vi "Configuration Parse.vi"(8 "error in":errorcluster, 11 "Measurement Configuration":T1={"Automation Test"=FALSE, "Power sequencing file path"="", "VST Resource Name"="5842", "RFSG port"="Port1", "RFmx port"="Port2", "RF Out Switch"="2599_S8", "Common RFout"="COM0", "Port1 Incident"="NC0", "Port2 Incident"="NO0", "RF In Switch"="2597_S12", "Common RFin"="COM", "Port1 Reference"="CH1", "Port1 Test"="CH2", "Port2 Reference"="CH4", "Port2 Test"="CH3", "RFSG attenuation mode"=enum."<None>", "RFSG external attenuation (dB)"=0.0, "Save Calibration File at"="", "Short S1P"="", "Open S1P"="", "Load S1P"="", "Through Adapter S2P"="", "Action"=enum."Measure", "Power Level (dBm)"=0.0, "External Gain (dB)"=-6.0, "Start Frequency (Hz)"=6000000000.0, "Stop Frequency (Hz)"=12000000000.0, "Step Size (Hz)"=100000000.0, "Type of Stimulus"=enum."CW", "Pulse Width (s)"=0.0, "PRI (s)"=0.0, "IF Bandwidth (Hz)"=10000.0, "Average Mode"=enum."Per Sweep", "Number of Averages"=1, "SnP File Path"="", "Calibration File Path"="", "Power sequecing file validity check"=TRUE} {"Step Size (Hz)" format="%#_6p"; "Stop Frequency (Hz)" format="%.3p"; "Start Frequency (Hz)" format="%.3p"; "Power Level (dBm)" format="%.2f"; "RFSG external attenuation (dB)" format="%.2f"}) -> (0 "error out":errorcluster, 2 "RFmxVNA Settings":T3={"VST Resource Name"="VNA-5633", "RFSG Port"="", "RFmx Port"="", "RF Out Switch"="VNA-5633", "RF Out Connection"={"Common RFout"="", "Port1 Incident"="", "Port2 Incident"=""}, "RF In Switch"="VNA-5633", "RF In Connection"={"Common RFin"="", "Port1 Reference"="", "Port1 Test"="", "Port2 Reference"="", "Port2 Test"=""}, "RFSG attenuation mode"=enum."Constant Attenuation", "RFSG Constant Attenuation (dB)"=0.0, "Save Calibration File at"=path "", "Short S1P"=path "", "Open S1P"=path "", "Load S1P"=path "", "Through Adapter S2P"=path ""}, 3 "Test Configuration":T2={"Action"=enum."Measure", "Power Level (dBm)"=0.0, "External Gain (dB)"=0.0, "Frequency Sweep"={"Start Frequency (Hz)"=0.0, "Stop Frequency (Hz)"=0.0, "Step Size (Hz)"=0.0}, "Type of Stimulus"=enum."CW", "Pulse Width (s)"=0.0, "PRI (s)"=0.0, "IF Bandwidth (Hz)"=0.0, "Average Mode"=enum."Per Sweep", "Number of Averages"=0, "SnP File Path"=path "", "Calibration File Path"=path ""} {"Frequency Sweep"."Step Size (Hz)" format="%#_6p"; "Frequency Sweep"."Stop Frequency (Hz)" format="%.3p"; "Frequency Sweep"."Start Frequency (Hz)" format="%.3p"})   [LabVIEW 2023, in "FPT_SParam_VST.lvclass"]
uses:
  FPT_SParam_VST.lvclass
  Measurement/Controls/Hardware Config - SParam_VST.ctl
  Measurement/Controls/Test Config - SParam_VST.ctl
  Measurement Configuration.ctl
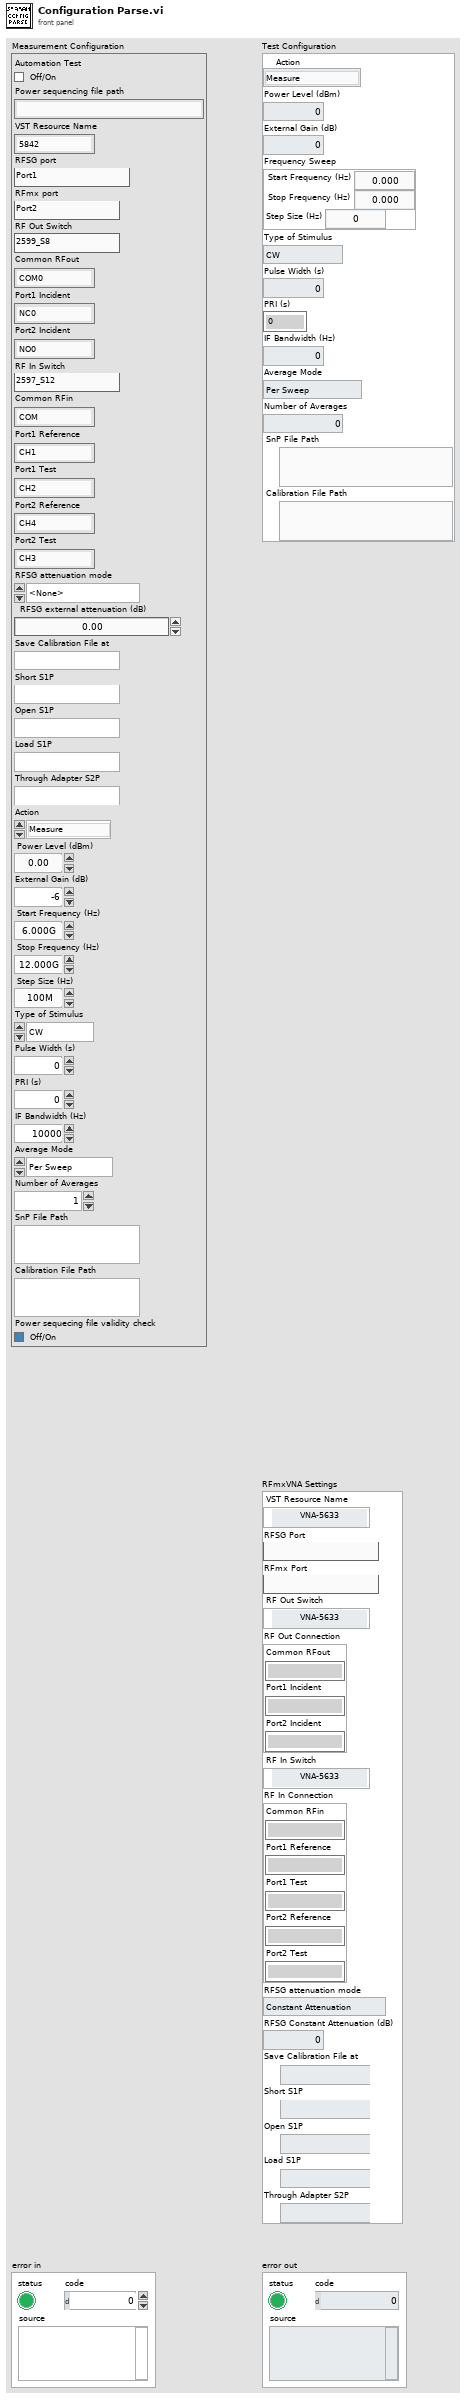
[diagram p1: front panel]
types:
  T1 = typedef "FPT_SParam_VST.lvclass/Measurement Configuration.ctl" = cluster{"Automation Test":bool, "Power sequencing file path":string, "VST Resource Name":string, "RFSG port":string, "RFmx port":string, "RF Out Switch":string, "Common RFout":string, "Port1 Incident":string, "Port2 Incident":string, "RF In Switch":string, "Common RFin":string, "Port1 Reference":string, "Port1 Test":string, "Port2 Reference":string, "Port2 Test":string, "RFSG attenuation mode":enum32{"<None>", "Constant Attenuation"}, "RFSG external attenuation (dB)":dbl, "Save Calibration File at":string, "Short S1P":string, "Open S1P":string, "Load S1P":string, "Through Adapter S2P":string, "Action":enum32{"Calibrate", "Measure"}, "Power Level (dBm)":dbl, "External Gain (dB)":dbl, "Start Frequency (Hz)":dbl, "Stop Frequency (Hz)":dbl, "Step Size (Hz)":dbl, "Type of Stimulus":enum32{"CW", "Pulsed CW"}, "Pulse Width (s)":dbl, "PRI (s)":dbl, "IF Bandwidth (Hz)":dbl, "Average Mode":enum32{"Per Sweep", "Per Point"}, "Number of Averages":i32, "SnP File Path":string, "Calibration File Path":string, "Power sequecing file validity check":bool}
  T2 = typedef "Test Config - SParam_VST.ctl" = cluster{"Action":enum32{"Calibrate", "Measure"}, "Power Level (dBm)":dbl, "External Gain (dB)":dbl, "Frequency Sweep":cluster{"Start Frequency (Hz)":dbl, "Stop Frequency (Hz)":dbl, "Step Size (Hz)":dbl}, "Type of Stimulus":enum16{"CW", "Pulsed CW"}, "Pulse Width (s)":dbl, "PRI (s)":dbl, "IF Bandwidth (Hz)":dbl, "Average Mode":enum16{"Per Sweep", "Per Point"}, "Number of Averages":i32, "SnP File Path":path, "Calibration File Path":path}
  T3 = typedef "Hardware Config - SParam_VST.ctl" = cluster{"VST Resource Name":refnum<k15>, "RFSG Port":string, "RFmx Port":string, "RF Out Switch":refnum<k15>, "RF Out Connection":cluster{"Common RFout":string, "Port1 Incident":string, "Port2 Incident":string}, "RF In Switch":refnum<k15>, "RF In Connection":cluster{"Common RFin":string, "Port1 Reference":string, "Port1 Test":string, "Port2 Reference":string, "Port2 Test":string}, "RFSG attenuation mode":enum32{"<None>", "Constant Attenuation"}, "RFSG Constant Attenuation (dB)":dbl, "Save Calibration File at":path, "Short S1P":path, "Open S1P":path, "Load S1P":path, "Through Adapter S2P":path}
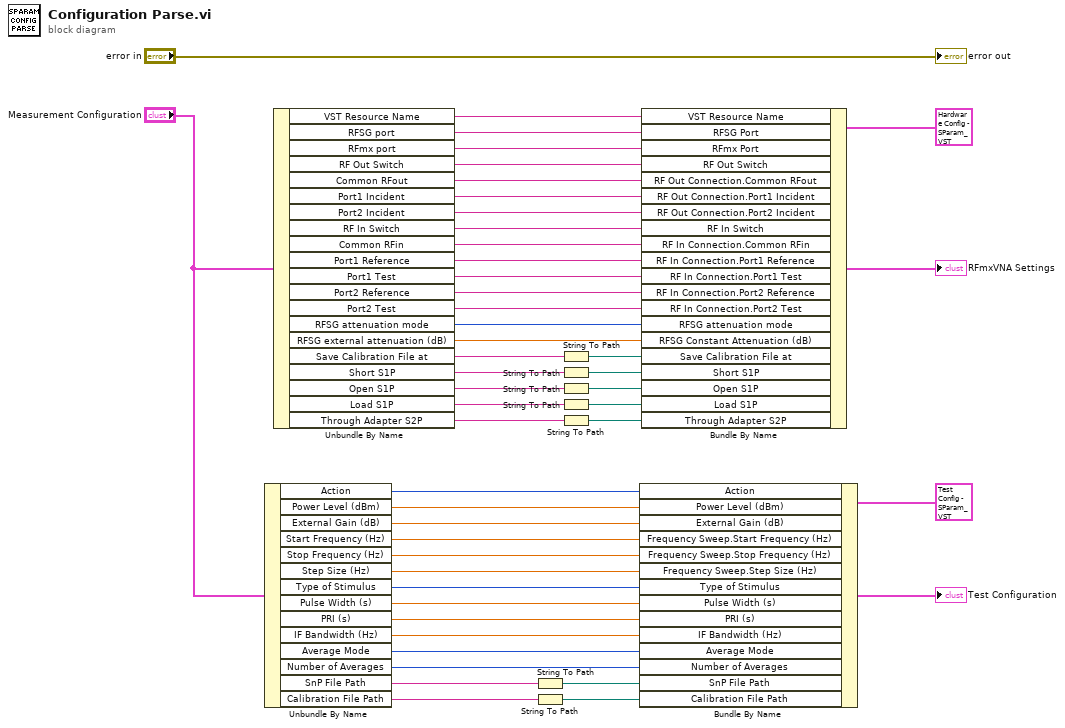
[diagram p0: block diagram]
diagram:
  n1 = Unbundle By Name("Measurement Configuration") -> ("Action"=w15:enum32{"Calibrate", "Measure"}, "Power Level (dBm)"=w16:dbl, "External Gain (dB)"=w14:dbl, "Start Frequency (Hz)"=w13:dbl, "Stop Frequency (Hz)"=w12:dbl, "Step Size (Hz)"=w11:dbl, "Type of Stimulus"=w10:enum32{"CW", "Pulsed CW"}, "Pulse Width (s)"=w9:dbl, "PRI (s)"=w8:dbl, "IF Bandwidth (Hz)"=w7:dbl, "Average Mode"=w6:enum32{"Per Sweep", "Per Point"}, "Number of Averages"=w5:i32, "SnP File Path"=w4:string, "Calibration File Path"=w2:string)
  n2 = Unbundle By Name("Measurement Configuration") -> ("VST Resource Name"=w41:string, "RFSG port"=w40:string, "RFmx port"=w39:string, "RF Out Switch"=w38:string, "Common RFout"=w37:string, "Port1 Incident"=w36:string, "Port2 Incident"=w35:string, "RF In Switch"=w34:string, "Common RFin"=w33:string, "Port1 Reference"=w32:string, "Port1 Test"=w31:string, "Port2 Reference"=w30:string, "Port2 Test"=w29:string, "RFSG attenuation mode"=w28:enum32{"<None>", "Constant Attenuation"}, "RFSG external attenuation (dB)"=w27:dbl, "Save Calibration File at"=w26:string, "Short S1P"=w24:string, "Open S1P"=w22:string, "Load S1P"=w20:string, "Through Adapter S2P"=w18:string)
  n3 = String To Path(string=w4) -> (path=w3:path)
  n4 = String To Path(string=w2) -> (path=w1:path)
  n5 = String To Path(string=w26) -> (path=w25:path)
  n6 = String To Path(string=w24) -> (path=w23:path)
  n7 = String To Path(string=w22) -> (path=w21:path)
  n8 = String To Path(string=w20) -> (path=w19:path)
  n9 = String To Path(string=w18) -> (path=w17:path)
  n10 = Bundle By Name(cluster=T2 {"Action"=enum."Measure", "Power Level (dBm)"=0.0, "External Gain (dB)"=0.0, "Frequency Sweep"={"Start Frequency (Hz)"=4000000000.0, "Stop Frequency (Hz)"=26000000000.0, "Step Size (Hz)"=200.0}, "Type of Stimulus"=enum."CW", "Pulse Width (s)"=0.0, "PRI (s)"=0.0, "IF Bandwidth (Hz)"=0.0, "Average Mode"=enum."Per Sweep", "Number of Averages"=0, "SnP File Path"=path "", "Calibration File Path"=path ""} ("Test Configuration"), "Action"=w15, "Power Level (dBm)"=w16, "External Gain (dB)"=w14, "Frequency Sweep.Start Frequency (Hz)"=w13, "Frequency Sweep.Stop Frequency (Hz)"=w12, "Frequency Sweep.Step Size (Hz)"=w11, "Type of Stimulus"=w10, "Pulse Width (s)"=w9, "PRI (s)"=w8, "IF Bandwidth (Hz)"=w7, "Average Mode"=w6, "Number of Averages"=w5, "SnP File Path"=w3, "Calibration File Path"=w1) -> (→"Test Configuration":T2)
  n11 = Bundle By Name(cluster=T3 {"VST Resource Name"="", "RFSG Port"="", "RFmx Port"="", "RF Out Switch"="", "RF Out Connection"={"Common RFout"="", "Port1 Incident"="", "Port2 Incident"=""}, "RF In Switch"="", "RF In Connection"={"Common RFin"="", "Port1 Reference"="", "Port1 Test"="", "Port2 Reference"="", "Port2 Test"=""}, "RFSG attenuation mode"=enum."<None>", "RFSG Constant Attenuation (dB)"=0.0, "Save Calibration File at"=path "", "Short S1P"=path "", "Open S1P"=path "", "Load S1P"=path "", "Through Adapter S2P"=path ""} ("RFmxVNA Settings"), "VST Resource Name"=w41, "RFSG Port"=w40, "RFmx Port"=w39, "RF Out Switch"=w38, "RF Out Connection.Common RFout"=w37, "RF Out Connection.Port1 Incident"=w36, "RF Out Connection.Port2 Incident"=w35, "RF In Switch"=w34, "RF In Connection.Common RFin"=w33, "RF In Connection.Port1 Reference"=w32, "RF In Connection.Port1 Test"=w31, "RF In Connection.Port2 Reference"=w30, "RF In Connection.Port2 Test"=w29, "RFSG attenuation mode"=w28, "RFSG Constant Attenuation (dB)"=w27, "Save Calibration File at"=w25, "Short S1P"=w23, "Open S1P"=w21, "Load S1P"=w19, "Through Adapter S2P"=w17) -> (→"RFmxVNA Settings":T3)
  "error out" <- "error in"
